vi "Format Key Name to String.vi"(10 "Key":string, 11 "Section":string) -> (3 "String out":string)   [LabVIEW 2018, in "Configuration File.lvlib" / "Configuration File.lvclass"]
doc: "This method takes in the key and section, and formats a string that represents it."
uses:
  Configuration File.lvclass
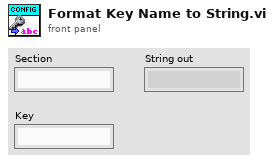
[diagram p1: front panel]
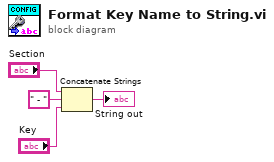
[diagram p0: block diagram]
diagram:
  n1 = Concatenate Strings("Section", " - " ("string"), "Key") -> (→"String out":string)
